vi "HS_RunScript.vi"(8 "error in":errorcluster, 9 "Console In":string, 10 "script":string, 11 "VISA Refnum in":refnum<visa-resource-name>) -> (0 "error out":errorcluster, 1 "Console Out":string, 2 "Tx":string, 3 "VISA Refnum out":refnum<visa-resource-name>)   [LabVIEW 2019]
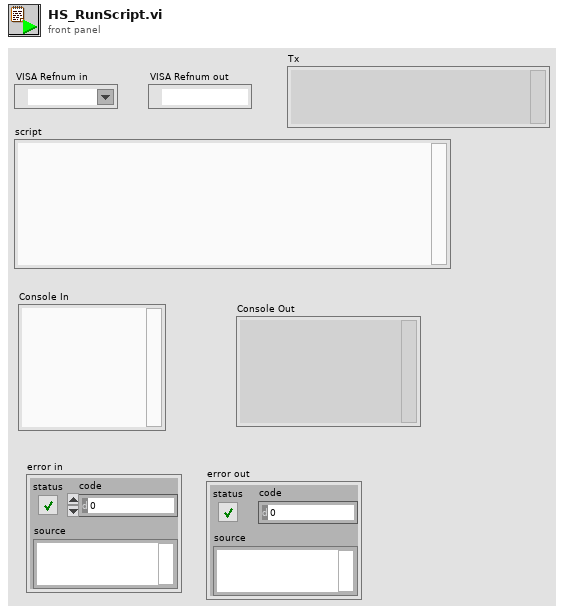
[diagram p1: front panel]
types:
  T1 = cluster{"Before":u8, "After":u8, "Send as 1 block?":bool}
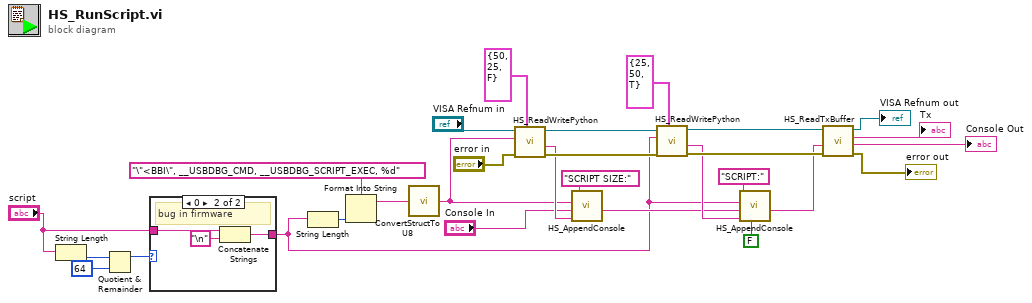
[diagram p0: block diagram]
diagram:
  n1 = String Length(string="script") -> (length=w7:i32)
  n2 = Quotient & Remainder(x=w7, y=64) -> (x-y*floor(x/y)=w5:i32)  [unwired: 1 out]
  n3 = case shown="0" w5 {
    tunnel: "script" -> [w30 w33]
    tunnel: [w30 w31] -> w3
    frame Default {
    }
    frame 0 {
      # "bug in firmware"
      n4 = Concatenate Strings(w33, "\n" ("string")) -> (w31:string)
    }
  }
  n5 = String Length(string=w3) -> (length=w28:i32)
  n6 = Format Into String(format string="\"<BBI\", __USBDBG_CMD, __USBDBG_SCRIPT_EXEC, %d" ("write buffer"), w28) -> (resulting string=w9:string)  [unwired: 2 in, 1 out]
  n7 = call <userlib>:"ConvertStructToU8.vi"("struct"=w9) -> ("Binary"=w8:string)
  n8 = call <userlib>:"HS_ReadWritePython.vi"("Timeouts (ms)"=T1 {"Before"=50, "After"=25, "Send as 1 block?"=FALSE}, "error in"="error in", "Write"=w8, "VISA in"="VISA Refnum in") -> ("error out"=w22:errorcluster, "Console Out"=w15:string, "VISA out"=w23:refnum<visa-resource-name>)  [unwired: 2 in, 3 out]
  n9 = call <userlib>:"HS_AppendConsole.vi"("Reply"=w15, "Console in"="Console In", "Send"=w8, "Command"="SCRIPT SIZE:") -> ("Console Out"=w14:string)  [unwired: 7 in]
  n10 = call <userlib>:"HS_ReadWritePython.vi"("Timeouts (ms)"=T1 {"Before"=25, "After"=50, "Send as 1 block?"=TRUE}, "error in"=w22, "Write"=w3, "VISA in"=w23) -> ("error out"=w21:errorcluster, "Console Out"=w16:string, "VISA out"=w20:refnum<visa-resource-name>)  [unwired: 2 in, 3 out]
  n11 = call <userlib>:"HS_AppendConsole.vi"("Show Send Binary?"=FALSE ("Show Binary?"), "Reply"=w16, "Console in"=w14, "Send"=w3, "Command"="SCRIPT:") -> ("Console Out"=w13:string)  [unwired: 6 in]
  n12 = call <userlib>:"HS_ReadTxBuffer.vi"("error in"=w21, "Console In"=w13, "VISA Refnum in"=w20) -> ("error out"=→"error out":errorcluster, "Console Out"=→"Console Out":string, "Tx Buffer"=→"Tx":string, "VISA Refnum out"=→"VISA Refnum out":refnum<visa-resource-name>)  [unwired: 5 in]
